vi "DigitalOscilloscope.vi"() -> ()   [LabVIEW 2014]
panel:
  in  "Digitizing Parameters":T1
  out "Waveform Graph":dbl[](graph)
  in  "stop":bool
  out "Numeric":dbl
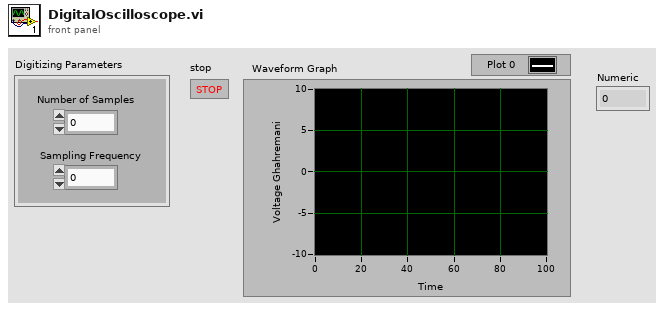
[diagram p1: front panel]
types:
  T1 = cluster{"Number of Samples":dbl, "Sampling Frequency":dbl}
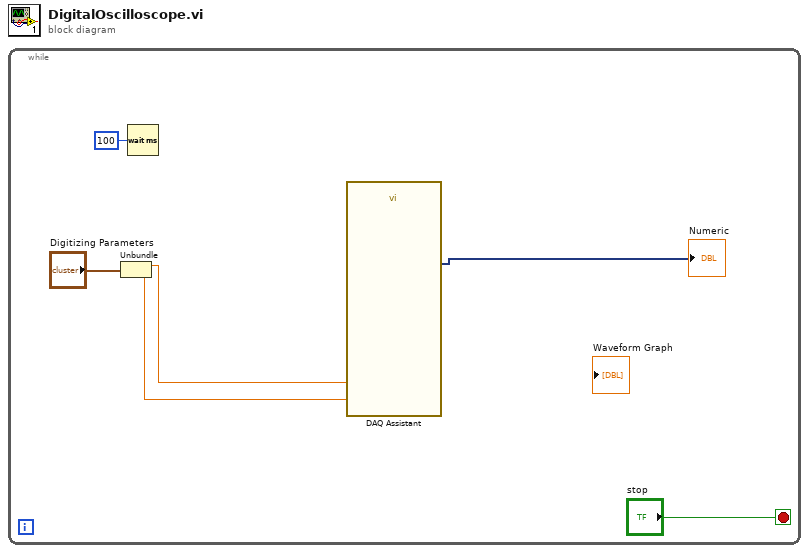
[diagram p0: block diagram]
diagram:
  n1 = while {
    stop <- "stop" stop-if-true
    n2 = Unbundle("Digitizing Parameters") -> ("Number of Samples"=w2:dbl, "Sampling Frequency"=w1:dbl)
    n3 = Wait (ms)(milliseconds to wait=u32 100) -> ()  [unwired: 1 out]
    n4 = call "DAQ Assistant"("rate"=w1, "number of samples"=w2) -> ("data"=→"Numeric":dynamicdata)  [unwired: 15 in, 2 out]
  }
